vi "Upload_To_ADAM_Server.vi"(1 "First Loop":bool, 2 "Averaging Period (s)":dbl=1.0, 3 "Shift In":dbl[](array[numeric]), 4 "Channel Values":dbl[](array[numeric]), 5 "Give Variance":bool, 6 "Channel Names":string[](array[string])) -> (0 "Shift Out":dbl[](array[numeric]))   [LabVIEW 2011]
uses:
  ADAM Controls/Update_scan_value.ctl
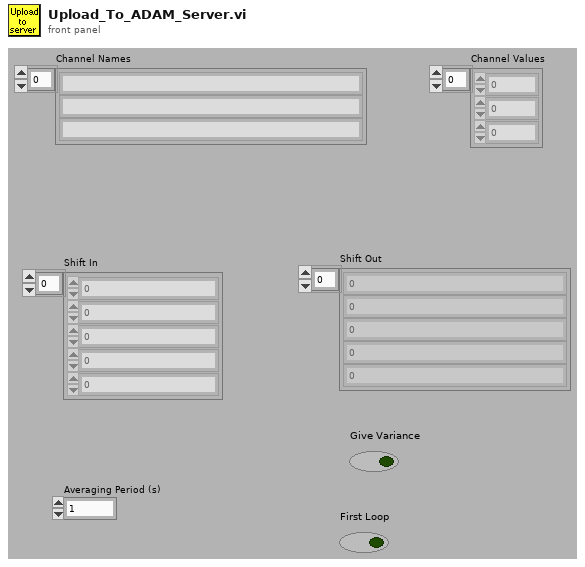
[diagram p1: front panel]
types:
  T1 = typedef "Update_scan_value.ctl" = cluster{"Channel Name":string, "New Value":dbl}
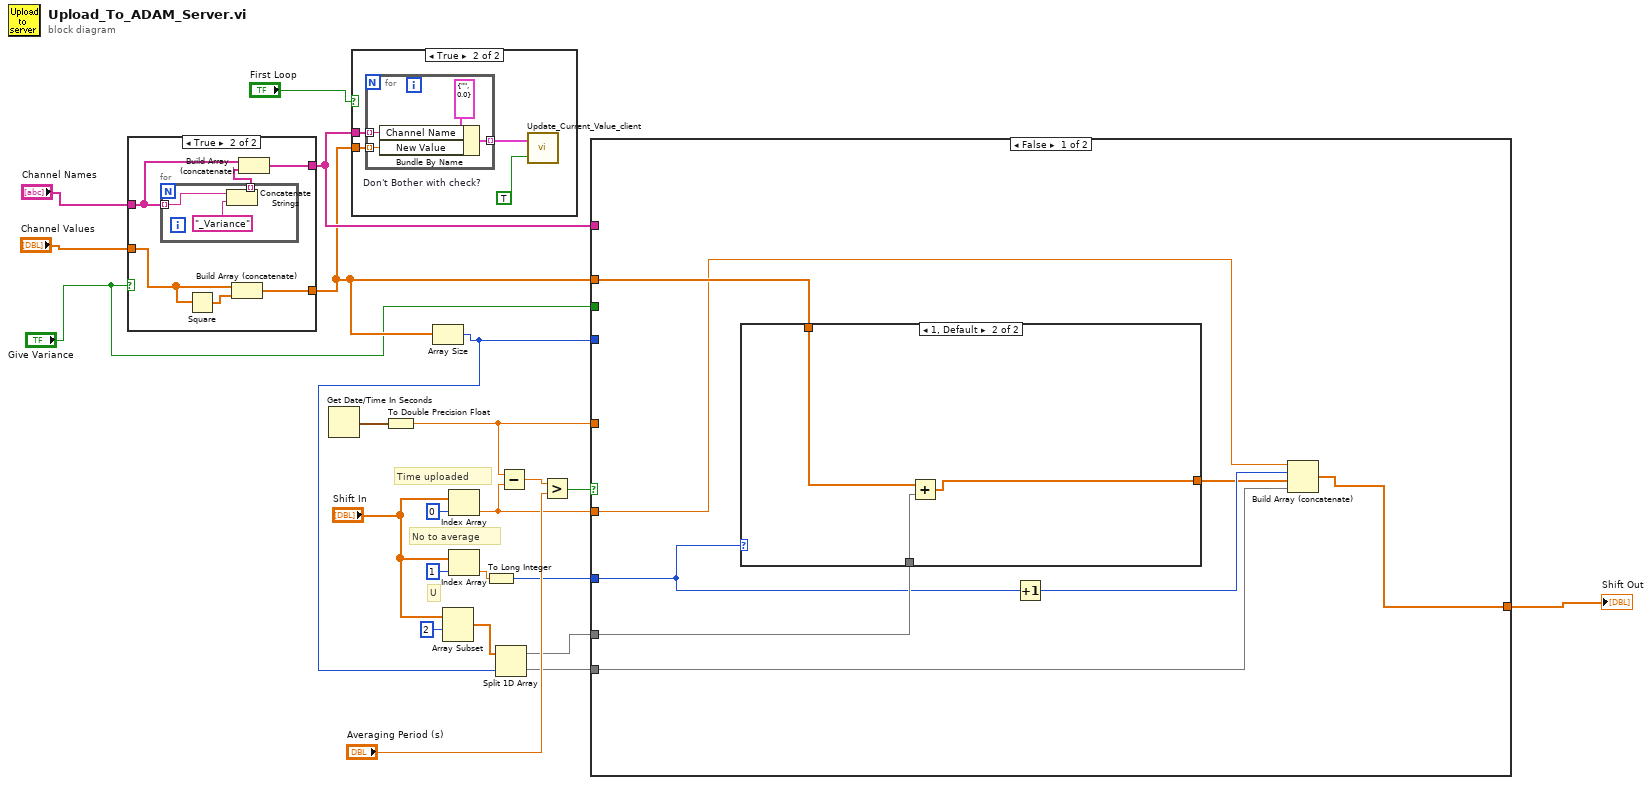
[diagram p0: block diagram]
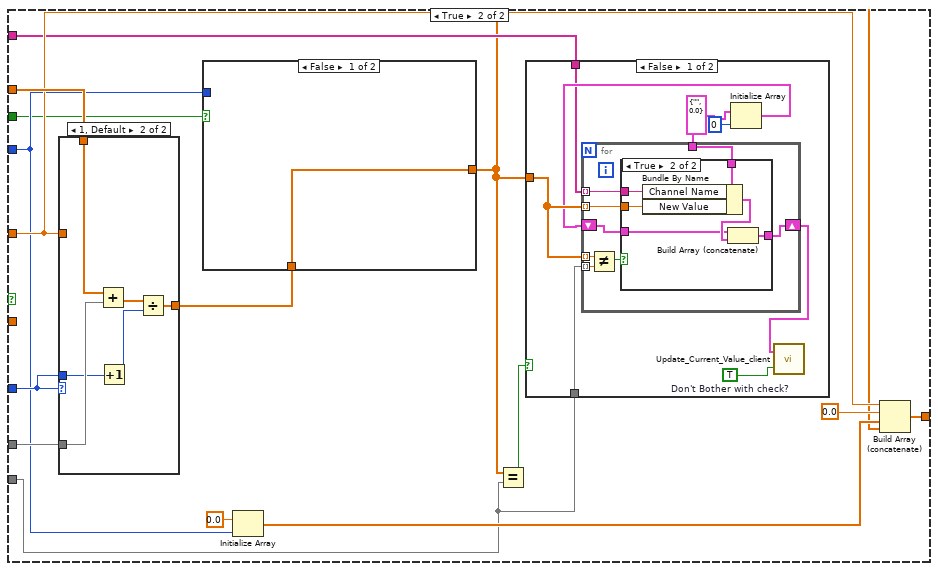
[diagram p5: hidden frame]
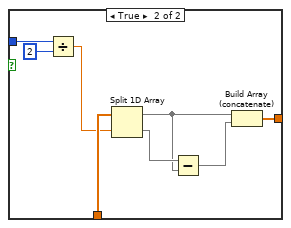
[diagram p6: hidden frame]
diagram:
  # "U"
  # "No to average"
  # "Time uploaded"
  n1 = case shown="True" "Give Variance" {
    tunnel: "Channel Names" -> [w25 w31]
    tunnel: [w25 w29] -> w4
    tunnel: "Channel Values" -> [w24 w27]
    tunnel: [w24 w26] -> w2
    frame False {
    }
    frame True {
      n2 = for {
        tunnel: w31 -> [w33] mode=indexing
        tunnel: [w32] -> w30 mode=indexing
        n3 = Concatenate Strings(w33, "_Variance") -> (w32:string)
      }
      n4 = Square(x=w27) -> (x^2=w28:dbl[])
      n5 = Build Array (concatenate)(w27, w28) -> (w26:dbl[])
      n6 = Build Array (concatenate)(w31, w30) -> (w29:string[])
    }
  }
  n7 = Get Date/Time In Seconds() -> (seconds since 1Jan1904=w22:timestamp)
  n8 = case shown="True" "First Loop" {
    tunnel: w4 -> [_ w36]
    tunnel: w2 -> [_ w35]
    frame False {
    }
    frame True {
      w38 = TRUE  # Don't Bother with check?
      n9 = for {
        tunnel: [w41] -> w37 mode=indexing
        tunnel: w36 -> [w40] mode=indexing
        tunnel: w35 -> [w39] mode=indexing
        n10 = Bundle By Name(cluster=T1 {"Channel Name"="", "New Value"=0.0} ("Update Scan Value Cluster"), "Channel Name"=w40, "New Value"=w39) -> (w41:T1)
      }
      n11 = call "Update_Current_Value_client.vi"("Don't Bother with check?"=w38, "Update array in"=w37) -> ()
    }
  }
  n12 = To Double Precision Float(number=w22) -> (double precision float=w13:dbl)
  n13 = Array Size(array=w2) -> (size(s)=w9:i32)
  n14 = Array Subset(array="Shift In", index=2) -> (w10:dbl[])  [unwired: 1 in]
  n15 = Index Array(array="Shift In", index=0) -> (element=w11:dbl)
  n16 = Index Array(array="Shift In", index=1) -> (element=w15:dbl)
  n17 = To Long Integer(number=w15) -> (32bit integer=w14:i32)
  n18 = Split 1D Array(array=w10, index=w9) -> (first subarray=w8:dbl[], second subarray=w7:dbl[])
  n19 = Subtract(x=w13, y=w11) -> (x-y=w21:dbl)
  n20 = Greater?(x=w21, y="Averaging Period (s)") -> (0:w19:bool)
  n21 = case shown="False" w19 {
    tunnel: w2 -> [w50 w69]
    tunnel: w8 -> [w49 w64]
    tunnel: w14 -> [w47 w68]
    tunnel: w13 -> [_ w67]
    tunnel: [w44 w65] -> w12
    tunnel: w11 -> [w48 _]
    tunnel: w9 -> [_ w58]
    tunnel: w7 -> [w43 w60]
    tunnel: w4 -> [_ w59]
    tunnel: "Give Variance" -> [_ w55]
    frame False {
      n22 = case shown="1, Default" w47 {
        tunnel: w50 -> [w51 w54]
        tunnel: w49 -> [_ w53]
        tunnel: [w51 w52] -> w45
        frame 0 {
        }
        frame 1, Default {
          n23 = Add(x=w54, y=w53) -> (x+y=w52:dbl[])
        }
      }
      n24 = Increment(x=w47) -> (x+1=w46:i32)
      n25 = Build Array (concatenate)(w48, w46, w45, w43) -> (w44:dbl[])
    }
    frame True {
      n26 = case shown="1, Default" w68 {
        tunnel: w67 -> [_ _]
        tunnel: w64 -> [_ w107]
        tunnel: w69 -> [w102 w108]
        tunnel: w68 -> [_ w106]
        tunnel: [w102 w103] -> w57
        frame 0 {
        }
        frame 1, Default {
          n27 = Add(x=w108, y=w107) -> (x+y=w105:dbl[])
          n28 = Increment(x=w106) -> (x+1=w104:i32)
          n29 = Divide(x=w105, y=w104) -> (x/y=w103:dbl[])
        }
      }
      n30 = case shown="False" w55 {
        tunnel: w58 -> [_ w78]
        tunnel: w57 -> [w70 w76]
        tunnel: [w70 w71] -> w56
        frame False {
        }
        frame True {
          n31 = Divide(x=w78, y=2) -> (x/y=w75:dbl)
          n32 = Split 1D Array(array=w76, index=w75) -> (first subarray=w73:dbl[], second subarray=w74:dbl[])
          n33 = Subtract(x=w74, y=w73) -> (x-y=w72:dbl[])
          n34 = Build Array (concatenate)(w73, w72) -> (w71:dbl[])
        }
      }
      n35 = Initialize Array(0.0 ("element"), w58) -> (w62:dbl[])
      n36 = Equal?(x=w56, y=w60) -> (x = y?=w61:bool)
      n37 = case shown="False" w61 {
        tunnel: w56 -> [w85 _]
        tunnel: w60 -> [w84 _]
        tunnel: w59 -> [w79 _]
        frame False {
          w86 = TRUE  # Don't Bother with check?
          w83 = T1 {"Channel Name"="", "New Value"=0.0} ("Update Scan Value Cluster")
          n38 = Initialize Array(w83, 0 ("dimension size")) -> (w81:T1[])
          n39 = for {
            tunnel: w83 -> [w94]
            tunnel: w79 -> [w93] mode=indexing
            tunnel: w85 -> [w92] mode=indexing
            shift-right: [w88] -> w80
            shift-left: w81 -> [w89]
            tunnel: w85 -> [w91] mode=indexing
            tunnel: w84 -> [w90] mode=indexing
            n40 = Not Equal?(x=w91, y=w90) -> (x != y?=w87:bool)
            n41 = case shown="True" w87 {
              tunnel: w94 -> [_ w101]
              tunnel: w93 -> [_ w100]
              tunnel: w92 -> [_ w99]
              tunnel: w89 -> [w95 w97]
              tunnel: [w95 w96] -> w88
              frame False {
              }
              frame True {
                n42 = Bundle By Name(cluster=w101, "Channel Name"=w100, "New Value"=w99) -> (w98:T1)
                n43 = Build Array (concatenate)(w97, w98) -> (w96:T1[])
              }
            }
          }
          n44 = call "Update_Current_Value_client.vi"("Don't Bother with check?"=w86, "Update array in"=w80) -> ()
        }
        frame True {
        }
      }
      n45 = Build Array (concatenate)(w67, 0.0 ("element"), w62, w56) -> (w65:dbl[])
    }
  }
  "Shift Out" <- w12
